vi "Convert dBV rms to dBm.vi"(8 "error in (no error)":errorcluster, 11 "Power Spectrum / PSD (dBV rms)":cluster{"f0":dbl, "df":dbl, "magnitude":dbl[]}) -> (0 "error out":errorcluster, 3 "Power Spectrum / PSD (dBm)":cluster{"f0":dbl, "df":dbl, "magnitude":dbl[]})   [LabVIEW 2017]
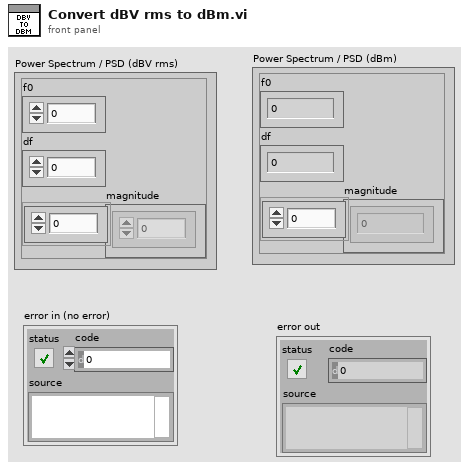
[diagram p1: front panel]
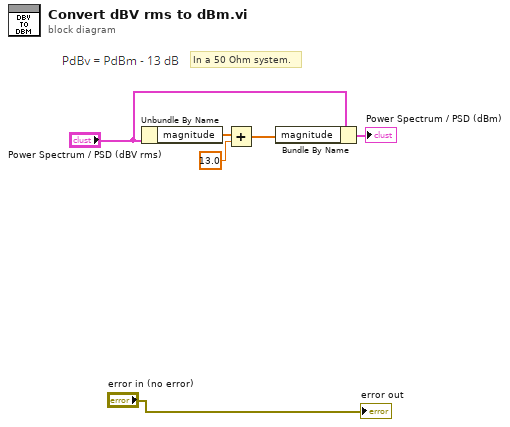
[diagram p0: block diagram]
diagram:
  # "In a 50 Ohm system."
  n1 = Unbundle By Name("Power Spectrum / PSD (dBV rms)") -> ("magnitude"=w6:dbl[])
  n2 = Add(x=w6, y=13.0) -> (x+y=w3:dbl[])
  n3 = Bundle By Name(cluster="Power Spectrum / PSD (dBV rms)", "magnitude"=w3) -> (→"Power Spectrum / PSD (dBm)":cluster{"f0":dbl, "df":dbl, "magnitude":dbl[]})
  "error out" <- "error in (no error)"
